vi "XBox 360 Controller.vi"() -> ()   [LabVIEW 2018]
uses:
  <vilib>/Utility/inputDevices.llb/joystickAcquire.vi
  <vilib>/Utility/inputDevices.llb/closeJoystick.vi
panel:
  in  "Zero TARGET":bool
  out "joystick info":T1(array[cluster])
  in  "SpinSpeed":dbl=65.0
  out "Target Angle":dbl(knob) scale=-180.0..180.0
  out "Y Coerced":dbl
  out "X Coerced":dbl
  in  "Tolerance":dbl=0.21
  out "Y axis Raw":dbl
  out "X axis Raw":dbl
  in  "stop":bool
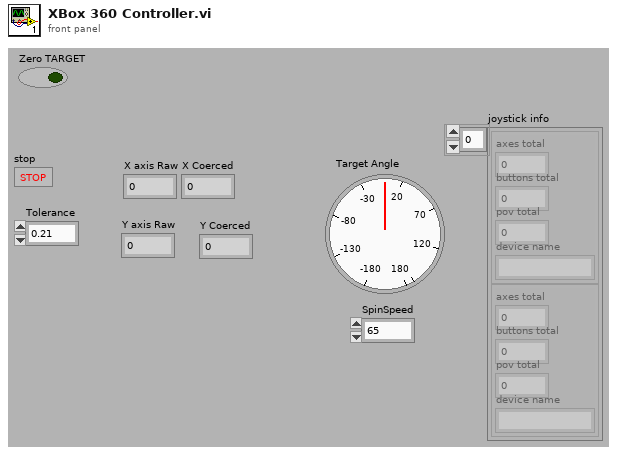
[diagram p1: front panel]
types:
  T1 = cluster{"axes total":u32, "buttons total":u32, "pov total":u32, "device name":string}[]
  T2 = cluster{"X axis":i32, "Y axis":i32, "Z axis":i32, "X axis rotation":i32, "Y axis rotation":i32, "Z axis rotation":i32, "U axis":i32, "V axis":i32}
  T3 = cluster{"button 1":bool, "button 2":bool, "button 3":bool, "button 4":bool, "button 5":bool, "button 6":bool, "button 7":bool, "button 8":bool, "button 9":bool, "button 10":bool, "button 11":bool, "button 12":bool, "button 13":bool, "button 14":bool, "button 15":bool, "button 16":bool, "button 17":bool, "button 18":bool, "button 19":bool, "button 20":bool, "button 21":bool, "button 22":bool, "button 23":bool, "button 24":bool, "button 25":bool, "button 26":bool, "button 27":bool, "button 28":bool, "button 29":bool, "button 30":bool, "button 31":bool, "button 32":bool}
  T4 = cluster{"pov 1":i32, "pov 2":i32, "pov 3":i32, "pov 4":i32}
  T5 = cluster{"Array[0]":bool, "Array[1]":bool, "Array[2]":bool, "Array[3]":bool, "Array[4]":bool, "Array[5]":bool, "Array[6]":bool, "Array[7]":bool, "Array[8]":bool}
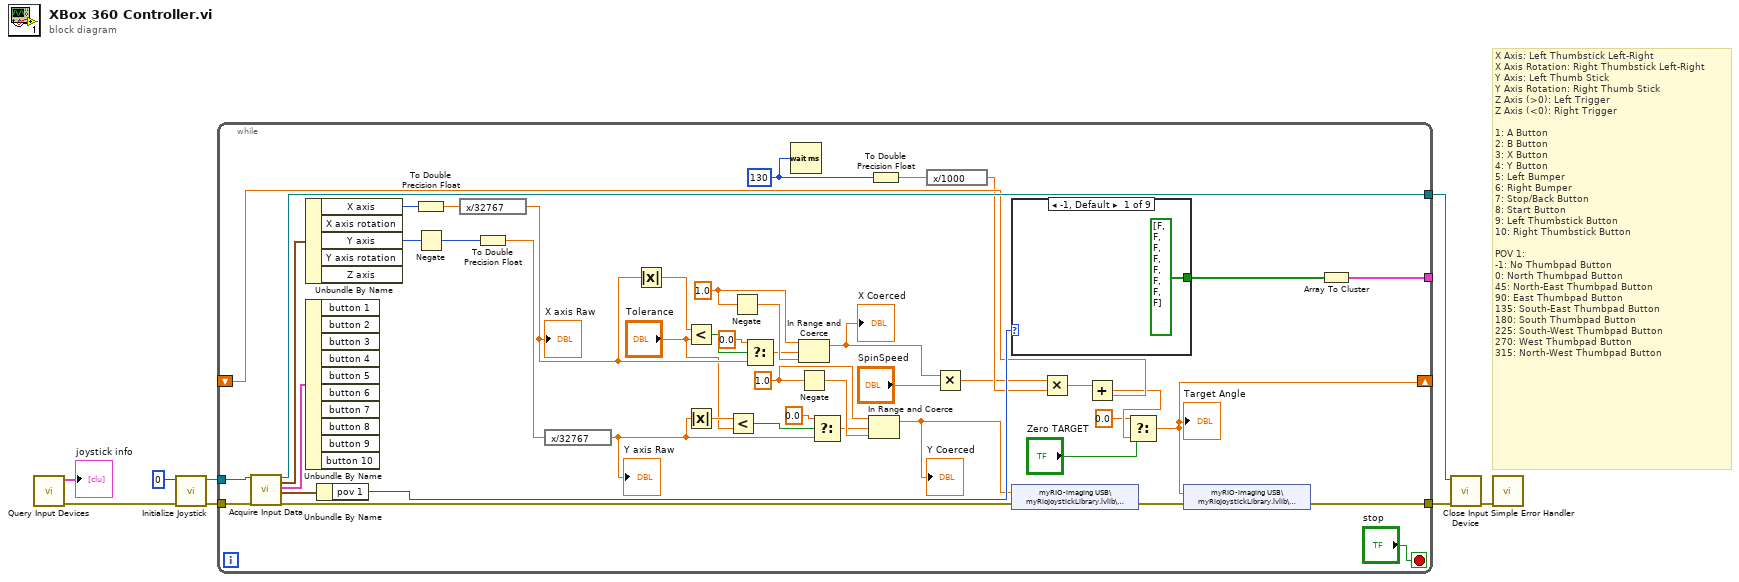
[diagram p0: block diagram]
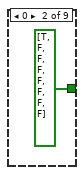
[diagram p2: hidden frame]
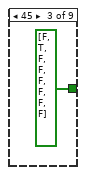
[diagram p3: hidden frame]
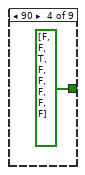
[diagram p4: hidden frame]
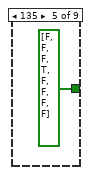
[diagram p5: hidden frame]
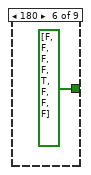
[diagram p6: hidden frame]
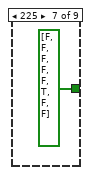
[diagram p7: hidden frame]
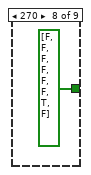
[diagram p8: hidden frame]
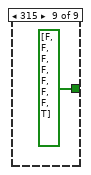
[diagram p9: hidden frame]
diagram:
  # "X Axis: Left Thumbstick Left-Right\nX Axis Rotation: Right Thumbstick Left-Right\nY Axis: Left Thumb Stick\nY Axis Rotation: Right Thumb Stick\nZ Axis (>0): Left Trigger\nZ Axis (<0): Right Trigger\n\n1: A Button\n2: B Button\n3: X Button\n4: Y Button\n5: Left Bumper\n6: Right Bumper\n7: Stop/Back Button\n8: Start Button\n9: Left Thumbstick Button\n10: Right Thumbstick Button\n\nPOV 1:\n-1: No Thumbpad Button\n0: North Thumbpad Button\n45: North-East Thumbpad Button\n90: East Thumbpad Button\n135: South-East Thumbpad Button\n180: South Thumbpad Button\n225: South-West Thumbpad Button\n270: West Thumbpad Button\n315: North-West Thumbpad Button"
  n1 = call <vilib>:"Query Input Devices.vi"() -> ("error out"=w8:errorcluster, "joystick info"=→"joystick info":T1)  [unwired: 1 in, 9 out]
  n2 = call <vilib>:"Initialize Joystick.vi"("error in (no error)"=w8, "device index"=0) -> ("error out"=w4:errorcluster, "device ID"=w6:refnum<k1>)  [unwired: 8 out]
  n3 = while {
    tunnel: w6 -> [w54]
    tunnel: [w52] -> w5
    tunnel: w4 -> [w53]
    tunnel: [w21] -> w3
    tunnel: [w48] -> _
    shift-right: [w11] -> _
    shift-left: _ -> [w20]
    stop <- "stop" stop-if-true
    w19 = u32 130 ("milliseconds to wait")
    w31 = 1.0 ("upper limit")
    w38 = 1.0 ("upper limit")
    n4 = call-poly <vilib>:"Acquire Input Data.vi"("device ID"=w54, "error in (no error)"=w53) -> ("device ID"=w52:refnum<k1>, "axis info"=w45:T2, "button info"=w47:T3, "direction info"=w51:T4, "error out"=w23:errorcluster)  [unwired: 13 out]
    n5 = Unbundle By Name(w45) -> ("X axis"=w44:i32, "Y axis"=w41:i32)  [unwired: 3 out]
    n6 = Unbundle By Name(w47) -> ()  [unwired: 10 out]
    n7 = Unbundle By Name(w51) -> ("pov 1"=w50:i32)
    n8 = To Double Precision Float(number=w44) -> (double precision float=w43:dbl)
    n9 = Negate(x=w41) -> (-x=w40:i32)
    n10 = expression code="x/32767"(w43) -> (w33:dbl)
    "X axis Raw" <- w33
    n11 = To Double Precision Float(number=w40) -> (double precision float=w42:dbl)
    n12 = expression code="x/32767"(w42) -> (w26:dbl)
    "Y axis Raw" <- w26
    n13 = Absolute Value(x=w33) -> (abs(x)=w34:dbl)
    n14 = Less?(x=w34, y="Tolerance") -> (x < y?=w36:bool)
    n15 = Absolute Value(x=w26) -> (abs(x)=w27:dbl)
    n16 = Less?(x=w27, y="Tolerance") -> (x < y?=w29:bool)
    n17 = Negate(x=w38) -> (-x=w39:dbl)
    n18 = Select(t=0.0, s=w36, f=w33) -> (s? t:f=w35:dbl)
    n19 = Wait (ms)(milliseconds to wait=w19) -> ()  [unwired: 1 out]
    n20 = In Range and Coerce(upper limit=w38, x=w35, lower limit=w39) -> (coerced(x)=w15:dbl)  [unwired: 1 out]
    "X Coerced" <- w15
    n21 = Negate(x=w31) -> (-x=w32:dbl)
    n22 = Select(t=0.0, s=w29, f=w26) -> (s? t:f=w28:dbl)
    n23 = In Range and Coerce(upper limit=w31, x=w28, lower limit=w32) -> (coerced(x)=w24:dbl)  [unwired: 1 out]
    "Y Coerced" <- w24
    n24 = To Double Precision Float(number=w19) -> (double precision float=w18:dbl)
    n25 = expression code="x/1000"(w18) -> (w17:dbl)
    n26 = Multiply(x=w15, y="SpinSpeed") -> (x*y=w13:dbl)
    n27 = case shown="-1, Default" w50 {
      tunnel: [bool[] [FALSE, FALSE, FALSE, FALSE, FALSE, FALSE, FALSE, FALSE] ("Array") bool[] [TRUE, FALSE, FALSE, FALSE, FALSE, FALSE, FALSE, FALSE] ("Array") bool[] [FALSE, TRUE, FALSE, FALSE, FALSE, FALSE, FALSE, FALSE] ("Array") bool[] [FALSE, FALSE, TRUE, FALSE, FALSE, FALSE, FALSE, FALSE] ("Array") bool[] [FALSE, FALSE, FALSE, TRUE, FALSE, FALSE, FALSE, FALSE] ("Array") bool[] [FALSE, FALSE, FALSE, FALSE, TRUE, FALSE, FALSE, FALSE] ("Array") bool[] [FALSE, FALSE, FALSE, FALSE, FALSE, TRUE, FALSE, FALSE] ("Array") bool[] [FALSE, FALSE, FALSE, FALSE, FALSE, FALSE, TRUE, FALSE] ("Array") bool[] [FALSE, FALSE, FALSE, FALSE, FALSE, FALSE, FALSE, TRUE] ("Array")] -> w49
      frame -1, Default {
      }
      frame 0 {
      }
      frame 45 {
      }
      frame 90 {
      }
      frame 135 {
      }
      frame 180 {
      }
      frame 225 {
      }
      frame 270 {
      }
      frame 315 {
      }
    }
    n28 = shared-variable "myRIO-imaging USB\\myRioJoystickLibrary.lvlib\\myRioJoystickY"(w24, error in=w23) -> (error out=w22:errorcluster)
    n29 = Multiply(x=w13, y=w17) -> (x*y=w16:dbl)
    n30 = Add(x=w16, y=w20) -> (x+y=w12:dbl)
    n31 = Select(t=0.0, s="Zero TARGET", f=w12) -> (s? t:f=w11:dbl)
    "Target Angle" <- w11
    n32 = shared-variable "myRIO-imaging USB\\myRioJoystickLibrary.lvlib\\myRioJoystickX"(w11, error in=w22) -> (error out=w21:errorcluster)
    n33 = Array To Cluster(array=w49) -> (cluster=w48:T5)
  }
  n34 = call-poly <vilib>:"Close Input Device.vi"("error in (no error)"=w3, "device ID"=w5) -> ("error out"=w7:errorcluster)  [unwired: 8 out]
  n35 = call <vilib>:"Simple Error Handler.vi"("error in (no error)"=w7) -> ()  [unwired: 1 in, 8 out]
